vi "Common Headers.vi"(8 "error in (no error)":errorcluster, 11 "Request in":refnum<class "Request.lvclass">) -> (0 "error out":errorcluster, 3 "Request out":refnum<class "Request.lvclass">)   [LabVIEW 2020, in "HTTP Utils.lvlib" / "Request.lvclass"]
uses:
  Request.lvclass
  Request.lvclass/Request.ctl
  Form Type.ctl
  HTTP Utils.lvlib
  lv-uri/URI/URI/URI.lvclass
  lv-uri/URI/URI.lvlib
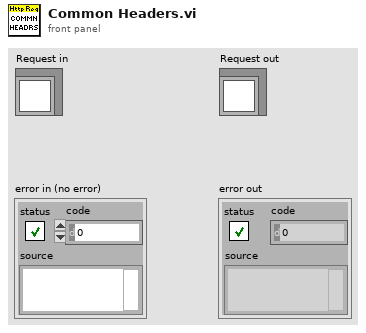
[diagram p1: front panel]
types:
  T1 = typedef "HTTP Utils.lvlib/Form Type.ctl" = enum16{"None", "UrlEncoded", "Multipart"}
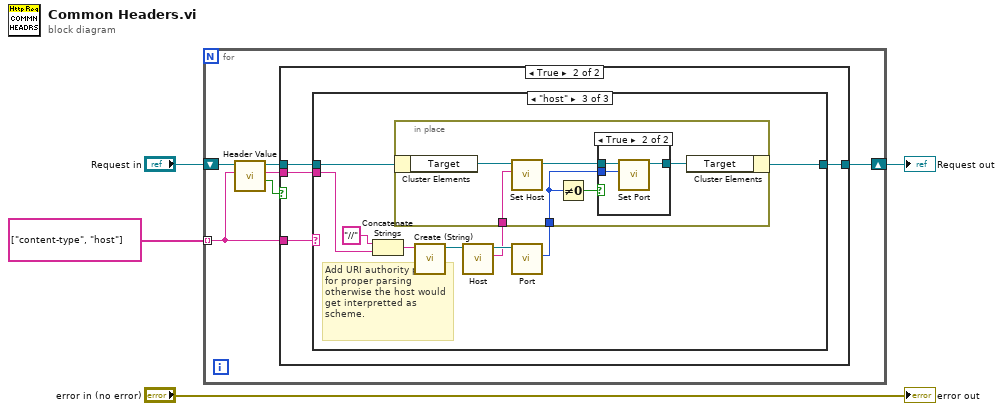
[diagram p0: block diagram]
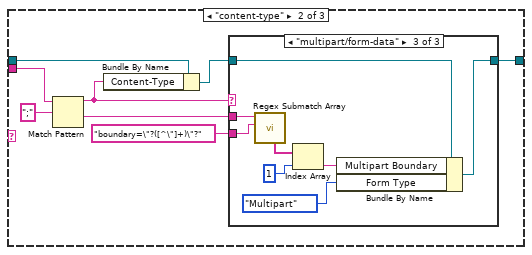
[diagram p4: hidden frame]
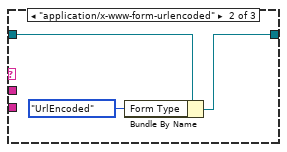
[diagram p6: hidden frame]
diagram:
  n1 = for {
    shift-right: [w7] -> w2
    shift-left: "Request in" -> [w10]
    tunnel: string[] ["content-type", "host"] -> [w5] mode=indexing
    n2 = call "Header Value.vi"("Header"=w5, "Request in"=w10) -> ("Exists"=w6:bool, "Value"=w8:string, "Request out"=w9:refnum<class "Request.lvclass">)  [unwired: 6 in, 1 out]
    n3 = case shown="True" w6 {
      tunnel: w9 -> [w11 w15]
      tunnel: w8 -> [_ w14]
      tunnel: [w11 w13] -> w7
      tunnel: w5 -> [_ w12]
      frame False {
      }
      frame True {
        n4 = case shown="\"host\"" w12 {
          tunnel: w15 -> [w16 w24 w40]
          tunnel: w14 -> [_ w23 w45]
          tunnel: [w16 w22 w37] -> w13
          frame Default {
          }
          frame "content-type" {
            n5 = Match Pattern(string=w23, regular expression=";") -> (before substring=w18:string, after substring=w17:string)  [unwired: 1 in, 2 out]
            n6 = Bundle By Name(cluster=w24, "Content-Type"=w18) -> (w20:refnum<class "Request.lvclass">)
            n7 = case shown="\"multipart/form-data\"" w18 {
              tunnel: w20 -> [w25 w28 w36]
              tunnel: [w25 w26 w35] -> w22
              tunnel: w17 -> [_ _ w34]
              tunnel: "boundary=\"?([^\"]+)\"?" ("regular expression") -> [_ _ w33]
              frame Default {
              }
              frame "application/x-www-form-urlencoded" {
                n8 = Bundle By Name(cluster=w28, "Form Type"=Form_Type."UrlEncoded") -> (w26:refnum<class "Request.lvclass">)
              }
              frame "multipart/form-data" {
                n9 = call "Regex Submatch Array.vi"("regular expression"=w33, "string"=w34) -> ("matches"=w32:string[])  [unwired: 5 in, 4 out]
                n10 = Index Array(array=w32, index=1) -> (element=w30:string)
                n11 = Bundle By Name(cluster=w36, "Multipart Boundary"=w30, "Form Type"=Form_Type."Multipart") -> (w35:refnum<class "Request.lvclass">)
              }
            }
          }
          frame "host" {
            # "Add URI authority prefix for proper parsing otherwise the host would get interpretted as scheme."
            n12 = Concatenate Strings("//" ("string"), w45) -> (w44:string)
            n13 = call "Create (String).vi"("URI String"=w44) -> ("URI out"=w42:refnum<class "URI.lvclass">)  [unwired: 9 in, 1 out]
            n14 = call "Host.vi"("URI in"=w42) -> ("Host"=w39:string, "URI out"=w41:refnum<class "URI.lvclass">)  [unwired: 9 in]
            n15 = call "Port.vi"("URI in"=w41) -> ("Port"=w38:u16)  [unwired: 8 in, 2 out]
            n16 = in-place {
              in-place-border: w39 -> [w50]
              in-place-border: w38 -> [w48]
              n17 = in-place-cluster #1(w40) -> ("Target"=w51:refnum<class "URI.lvclass">)
              n18 = call "Set Host.vi"("Host"=w50, "URI in"=w51) -> ("URI out"=w49:refnum<class "URI.lvclass">)  [unwired: 9 in]
              n19 = Not Equal To 0?(x=w48) -> (x != 0?=w47:bool)
              n20 = case shown="True" w47 {
                tunnel: w49 -> [w52 w55]
                tunnel: w48 -> [_ w54]
                tunnel: [w52 w53] -> w46
                frame False {
                }
                frame True {
                  n21 = call "Set Port.vi"("Port"=w54, "URI in"=w55) -> ("URI out"=w53:refnum<class "URI.lvclass">)  [unwired: 9 in]
                }
              }
              n22 = in-place-cluster #1("Target"=w46) -> (w37:refnum<class "Request.lvclass">)
            }
          }
        }
      }
    }
  }
  "Request out" <- w2
  "error out" <- "error in (no error)"
